vi "Calculateur_Destination.vi"(8 "Error In":errorcluster caption="Entrée d'erreur", 11 "Donnees_Globales_IN":T1) -> (0 "Error Out":errorcluster, 3 "Donnees_Globale_Out":T1)   [LabVIEW 2019]
uses:
  Asc_State_Inputs.ctl
  Etat_Asc.ctl
panel:
  out "Etage_Actuel":i32
  out "Etage CIBLE":i32
  out "tABLEAU INF":bool[](array[boolean])
  out "tABLEAU SUP":bool[](array[boolean])
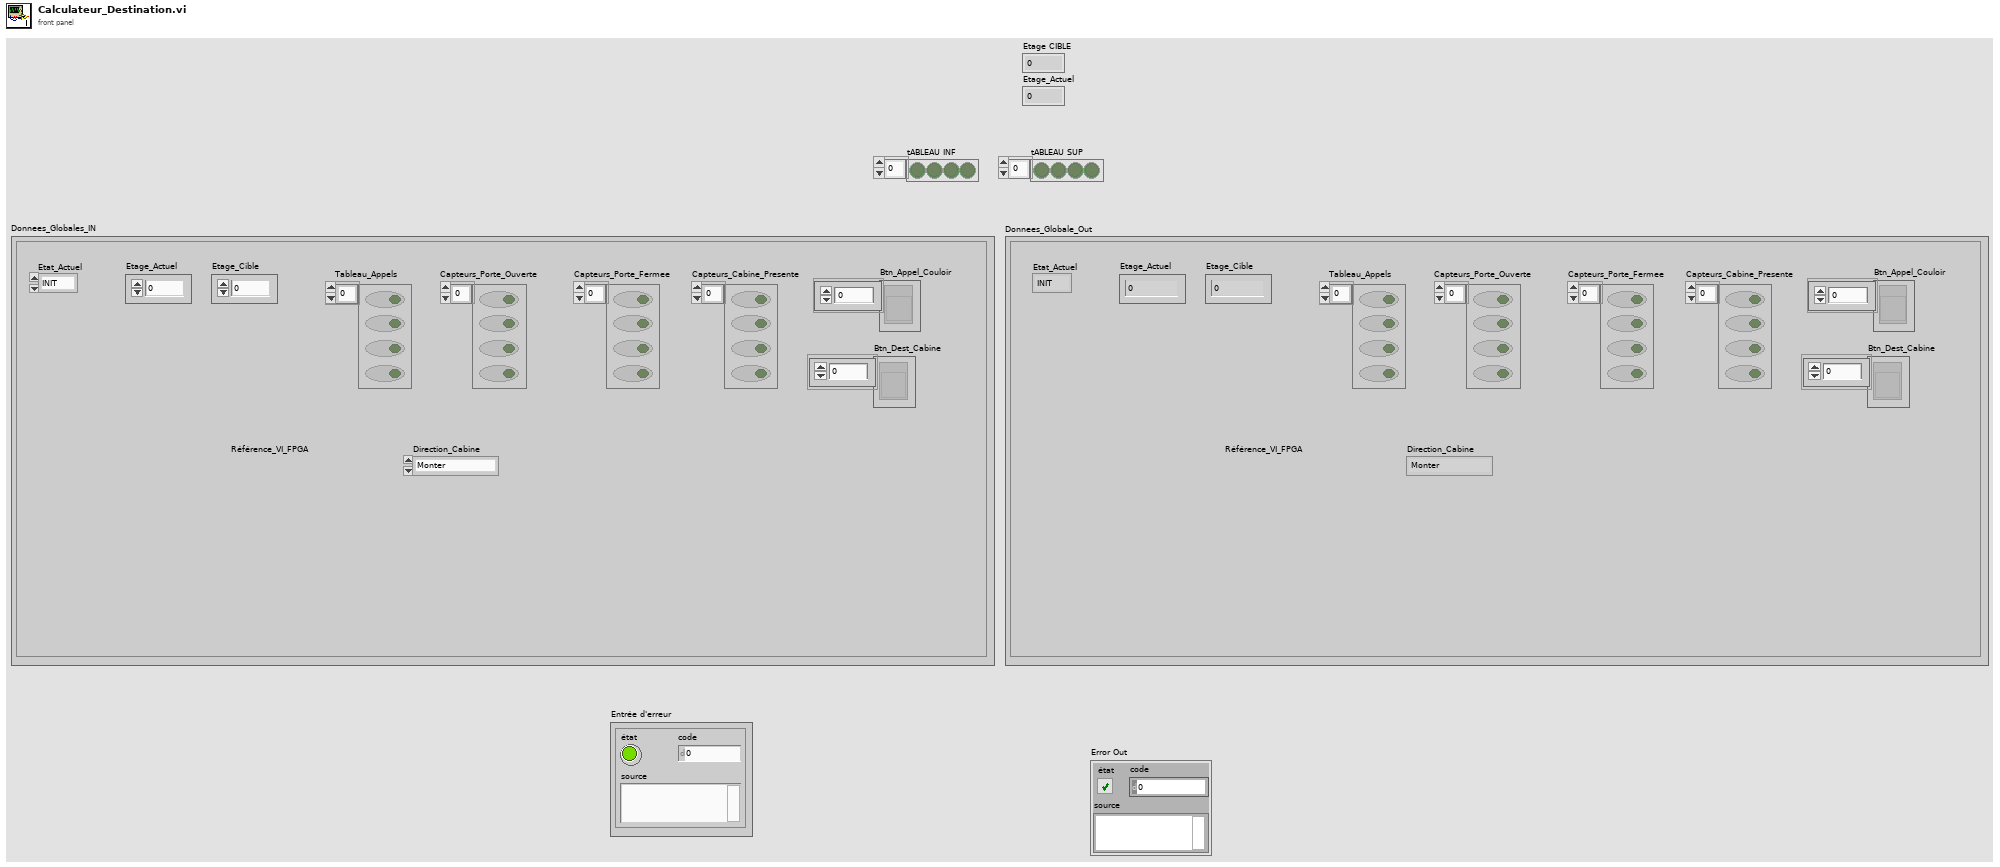
[diagram p1: front panel]
types:
  T1 = typedef "Asc_State_Inputs.ctl" = cluster{"Etage_Actuel":i32, "Etat_Actuel":T2, "Etage_Cible":i32, "Tableau_Appels":bool[], "Capteurs_Porte_Ouverte":bool[], "Capteurs_Porte_Fermee":bool[], "Capteurs_Cabine_Presente":bool[], "Btn_Appel_Couloir":refnum<vi>[], "Btn_Dest_Cabine":refnum<vi>[], "Référence_VI_FPGA":refnum<k20>, "Direction_Cabine":enum16{"Monter", "Descendre", "Arreter"}}
  T2 = typedef "Etat_Asc.ctl" = enum16{"INIT", "REPOS", "DEPLACEMENT", "OUVERTURE_PORTE", "ATTENTE_TEMPO", "FERMETURE_PORTE", "ARRET_URGENCE"}
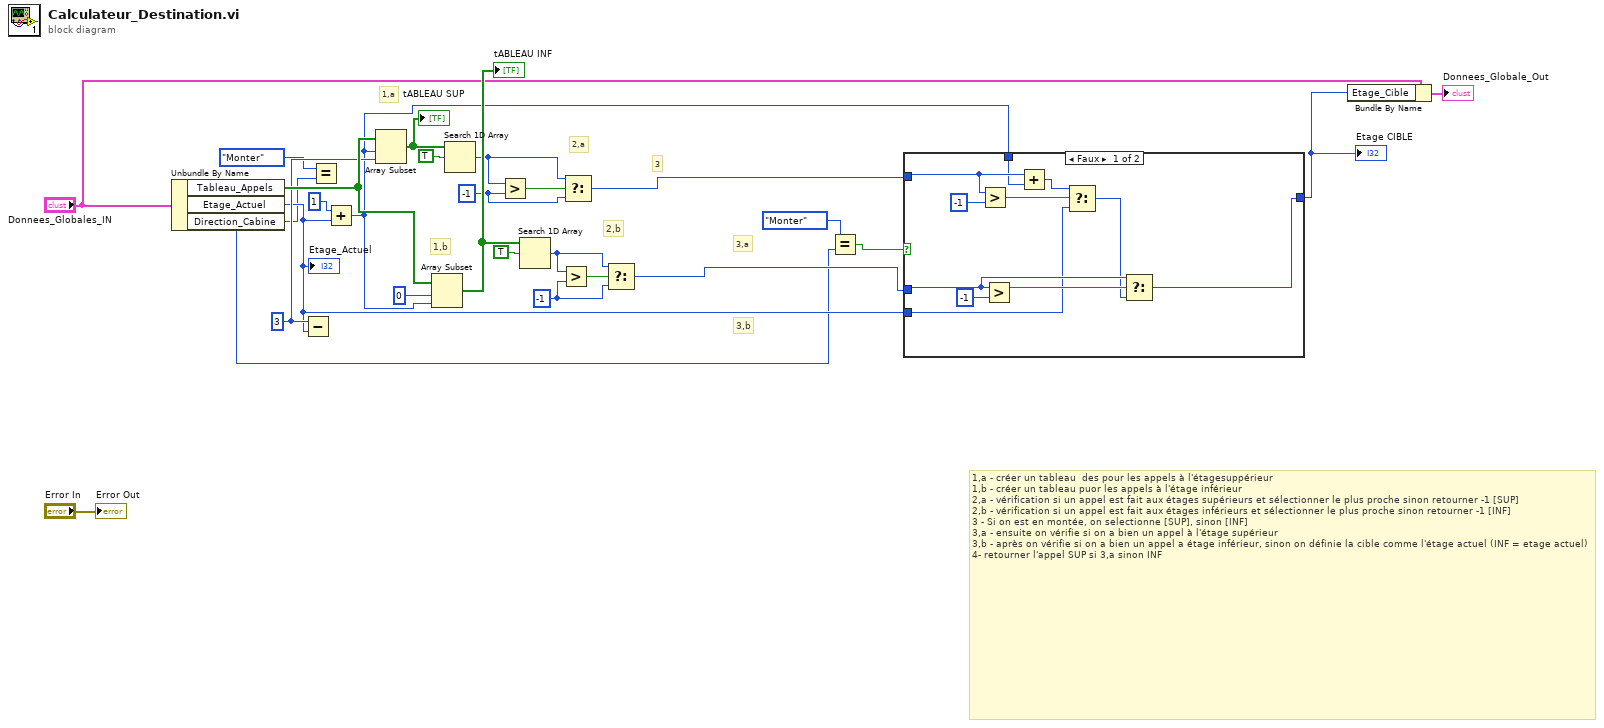
[diagram p0: block diagram]
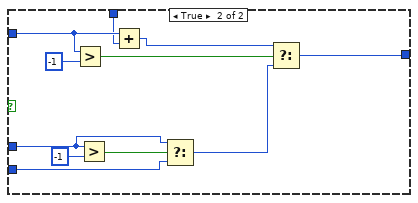
[diagram p2: hidden frame]
diagram:
  w11 = -1 ("y")
  w12 = -1 ("y")
  w21 = 3 ("longueur")
  # "3,b"
  # "3,a"
  # "3"
  # "2,b"
  # "2,a"
  # "1,b"
  # "1,a - créer un tableau  des pour les appels à l'étagesuppérieur\n1,b - créer un tableau puor les appels à l'étage inférieur\n2,a - vérification si un appel est fait aux étages supérieurs et sélectionner le plus proche sinon retourner -1 [SUP]\n2,b - vérification si un appel est fait aux étages inférieurs et sélectionner le plus proche sinon retourner -1 [INF]\n3 - Si on est en montée, on selectionne [SUP], sinon [INF]\n3,a - ensuite on vérifie si on a bien un appel à l'étage supérieur\n3,b - après on vérifie si on a bien un appel a étage inférieur, sinon on définie la cible comme l'étage actuel (INF = etage actuel)\n4- retourner l'appel SUP si 3,a sinon INF"
  # "1,a"
  n1 = Unbundle By Name("Donnees_Globales_IN") -> ("Tableau_Appels"=w25:bool[], "Etage_Actuel"=w5:i32, "Direction_Cabine"=w3:enum16{"Monter", "Descendre", "Arreter"})
  "Etage_Actuel" <- w5
  n2 = Subtract(x=w21, y=w5) -> ()  [unwired: 1 out]
  n3 = Equal?(x=enum16{"Monter", "Descendre", "Arreter"}."Monter" ("Direction_Cabine"), y=w3) -> ()  [unwired: 1 out]
  n4 = Add(x=1, y=w5) -> (x+y=w6:i32)
  n5 = Array Subset(array=w25, index=w6, length=w21) -> (w23:bool[])
  "tABLEAU SUP" <- w23
  n6 = Array Subset(array=w25, index=0 ("indice"), length=w6) -> (w22:bool[])
  "tABLEAU INF" <- w22
  n7 = Search 1D Array(1D array=w23, element=TRUE ("élément")) -> (index of element=w9:i32)  [unwired: 1 in]
  n8 = Greater?(x=w9, y=w12) -> (0:w10:bool)
  n9 = Search 1D Array(1D array=w22, element=TRUE ("élément")) -> (index of element=w17:i32)  [unwired: 1 in]
  n10 = Greater?(x=w17, y=w11) -> (0:w18:bool)
  n11 = Select(t=w9, s=w10, f=w12) -> (s? t:f=w8:i32)
  n12 = Select(t=w17, s=w18, f=w11) -> (s? t:f=w7:i32)
  n13 = Equal?(x=enum16{"Monter", "Descendre", "Arreter"}."Monter", y=w3) -> (x = y?=w1:bool)
  n14 = case shown="Faux" w1 {
    tunnel: w8 -> [w31 w45]
    tunnel: w7 -> [w32 w40]
    tunnel: [w30 w46] -> w4
    tunnel: w6 -> [w27 w44]
    tunnel: w5 -> [w29 w39]
    frame False {
      n15 = Greater?(x=w31, y=-1) -> (0:w36:bool)
      n16 = Greater?(x=w32, y=-1) -> (0:w33:bool)
      n17 = Add(x=w31, y=w27) -> (x+y=w35:i32)
      n18 = Select(t=w35, s=w36, f=w29) -> (s? t:f=w28:i32)
      n19 = Select(t=w32, s=w33, f=w28) -> (s? t:f=w30:i32)
    }
    frame True {
      n20 = Greater?(x=w45, y=-1) -> (0:w47:bool)
      n21 = Greater?(x=w40, y=-1) -> (0:w41:bool)
      n22 = Add(x=w45, y=w44) -> (x+y=w43:i32)
      n23 = Select(t=w40, s=w41, f=w39) -> (s? t:f=w38:i32)
      n24 = Select(t=w43, s=w47, f=w38) -> (s? t:f=w46:i32)
    }
  }
  "Etage CIBLE" <- w4
  n25 = Bundle By Name(cluster="Donnees_Globales_IN", "Etage_Cible"=w4) -> (→"Donnees_Globale_Out":T1)
  "Error Out" <- "Error In"
